vi "Create Temp DVR VI.vi"(8 "error in (no error)":errorcluster, 11 "DataValRefNum in":refnum<vi>) -> (0 "error out":errorcluster)   [LabVIEW 2018]
uses:
  <vilib>/Utility/traverseref.llb/TRef TravTarget.ctl
  <vilib>/Utility/miscctls.llb/LVPointTypeDef.ctl
  <vilib>/Utility/traverseref.llb/VI Scripting - Traverse.lvlib
panel:
  out "data":refnum<vi>[](array[refnum])
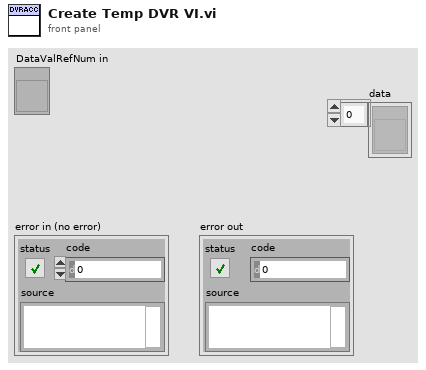
[diagram p1: front panel]
types:
  T1 = enum8{"Probe", "Diagram", "Panel Control", "3D Panel Control", "Dialog Panel Control", "Panel Indicator", "3D Panel Indicator", "Dialog Panel Indicator", "Power PC Control", "Power PC Indicator", "Silver Control", "Silver Indicator", "NXG Style Control", "NXG Style Indicator"}
  T2 = typedef "LVPointTypeDef.ctl" = cluster{"Horizontal":i16, "Vertical":i16}
  T3 = typedef "TRef TravTarget.ctl" = enum16{"FP", "BD", "Other"}
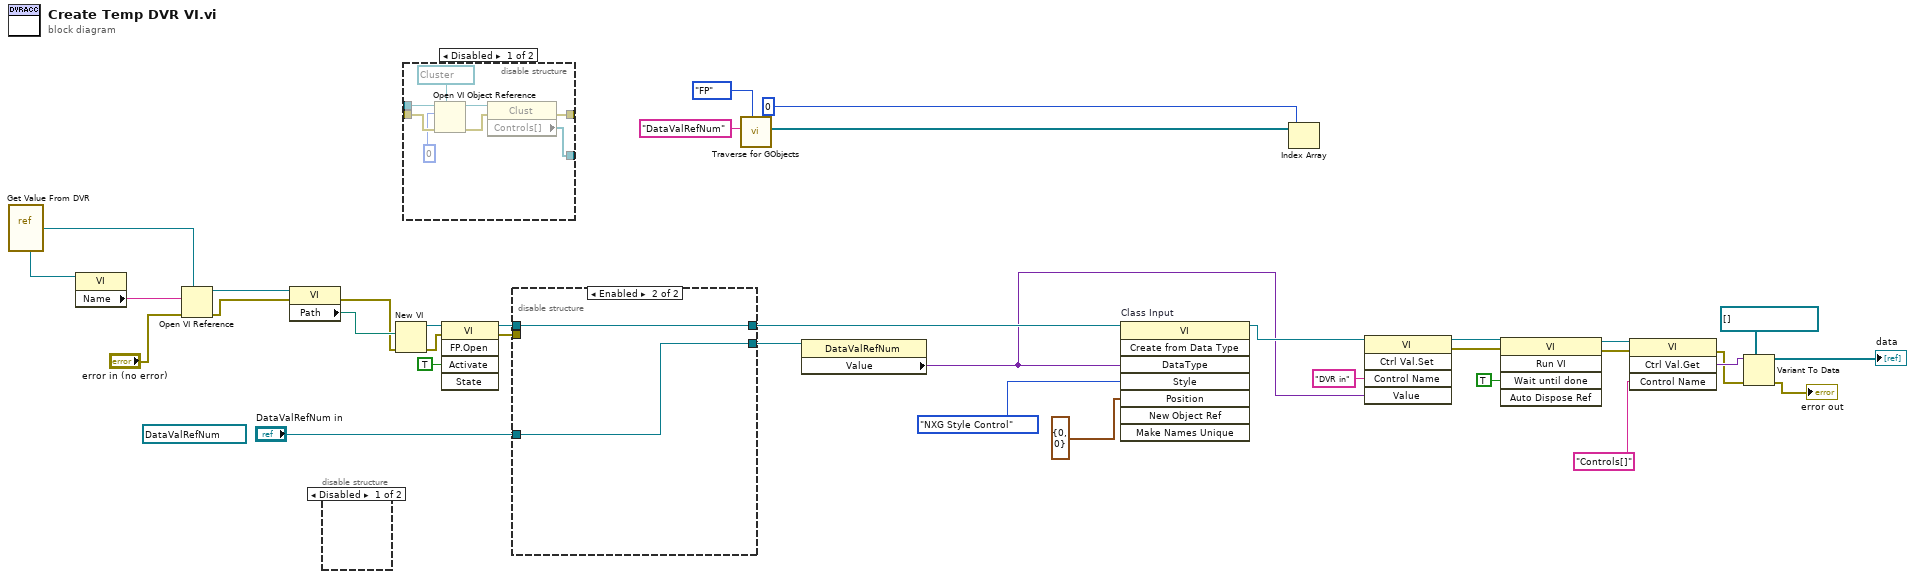
[diagram p0: block diagram]
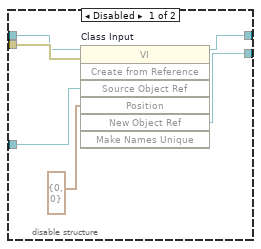
[diagram p2: hidden frame]
diagram:
  (unwired) refnum<vi> refnum ("DataValRefNum in")
  n1 = vi-ref "Get Value From DVR.vi"() -> (w24:refnum<vi>)
  n2 = property class="VI"(reference=w24) -> ("Name"=w25:string)  [unwired: 1 in, 2 out]
  n3 = Open VI Reference(type specifier VI Refnum (for type only)=w24, vi path=w25, error in (no error)="error in (no error)") -> (vi reference=w30:refnum<vi>, error out=w27:errorcluster)  [unwired: 3 in]
  n4 = property class="VI"(reference=w30, error in=w27) -> (error out=w26:errorcluster, "Path"=w29:path)  [unwired: 1 out]
  n5 = disable-structure shown="Disabled" {
    frame Disabled {
    }
    frame Enabled {
    }
  }
  n6 = New VI(8:w26, 10:w29) -> (0:w32:errorcluster, 3:w33:refnum<vi>)  [unwired: 5 in]
  n7 = disable-structure shown="Disabled" {
    disable-tunnel: [w43 _] -> _
    disable-tunnel: _ -> [w41 _]
    disable-tunnel: [w40 _] -> _
    disable-tunnel: _ -> [w37 _]
    frame Disabled {
      n8 = Open VI Object Reference(7:refnum<vi> refnum ("Numeric"), 8:w41, 10:0, 11:w37) -> (0:w42:errorcluster, 3:w39:refnum<vi>)
      n9 = property class="Clust"(reference=w39, error in=w42) -> (error out=w43:errorcluster, "Controls[]"=w40:refnum<vi>[])  [unwired: 1 out]
    }
    frame Enabled {
    }
  }
  n10 = invoke class="VI" method="FP.Open"(reference=w33, error in=w32, "Activate"=TRUE ("Activate?")) -> (reference out=w34:refnum<vi>, error out=w35:errorcluster)  [unwired: 2 in, 3 out]
  n11 = disable-structure shown="Enabled" {
    disable-tunnel: w35 -> [w49 _]
    disable-tunnel: w34 -> [w48 w51]
    disable-tunnel: "DataValRefNum in" -> [w47 w50]
    disable-tunnel: [w45 w50] -> w2
    disable-tunnel: [w44 w51] -> w4
    frame Disabled {
      n12 = invoke on="Class Input" class="VI" method="Create from Reference"(reference=w48, error in=w49, "Source Object Ref"=w47, "Position"=T2 {"Horizontal"=0, "Vertical"=0}) -> (reference out=w44:refnum<vi>, "New Object Ref"=w45:refnum<vi>)  [unwired: 3 in, 5 out]
    }
    frame Enabled {
    }
  }
  n13 = call <vilib>:"Traverse for GObjects.vi"("Traverse Target"=TRef_TravTarget."FP", "Class Name"="DataValRefNum") -> ("References"=w8:refnum<vi>[])  [unwired: 6 in, 3 out]
  n14 = property class="DataValRefNum"(reference=w2) -> ("Value"=w1:variant)  [unwired: 1 in, 2 out]
  n15 = invoke on="Class Input" class="VI" method="Create from Data Type"(reference=w4, "DataType"=w1, "Style"=T1."NXG Style Control", "Position"=T2 {"Horizontal"=0, "Vertical"=0}) -> (reference out=w3:refnum<vi>)  [unwired: 4 in, 7 out]
  n16 = Index Array(array=w8, index=0) -> ()  [unwired: 1 out]
  n17 = invoke class="VI" method="Ctrl Val.Set"(reference=w3, "Control Name"="DVR in", "Value"=w1) -> (reference out=w22:refnum<vi>, error out=w14:errorcluster)  [unwired: 2 in, 3 out]
  n18 = invoke class="VI" method="Run VI"(reference=w22, error in=w14, "Wait until done"=TRUE ("Wait Until Done")) -> (reference out=w20:refnum<vi>, error out=w19:errorcluster)  [unwired: 2 in, 3 out]
  n19 = invoke class="VI" method="Ctrl Val.Get"(reference=w20, error in=w19, "Control Name"="Controls[]") -> (error out=w13:errorcluster, "Get Control Value Variant"=w17:variant)  [unwired: 1 in, 2 out]
  n20 = Variant To Data(error in=w13, type=refnum<vi>[] [] ("Controls[]"), Variant=w17) -> (data=→"data":refnum<vi>[], error out=→"error out":errorcluster)
